vi "SRV_Write-Read Package.vi"(6 "Method":T2, 7 "parameters":T1={"bytes to read"=2000, "msec pause"=0, "msec timeout"=1000}, 8 "error in":errorcluster, 9 "listing in":string, 10 "data in":string, 11 "connection ID in":refnum<k5>) -> (0 "error out":errorcluster, 1 "listing out":string, 2 "data out":string, 3 "connection ID":refnum<k5>)   [LabVIEW 2014]
doc: "Modified for Benilde St. Margaret's School - Tim Jump\nBy Doug Schmertman - Logic PD\nCopyright 2012"
uses:
  SRV_Package Methods.ctl
  SRV_TCP Settings.ctl
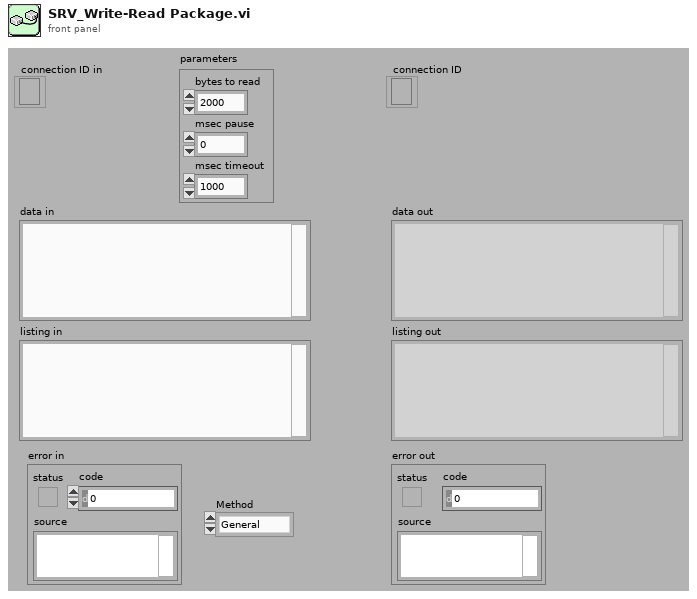
[diagram p1: front panel]
types:
  T1 = cluster{"bytes to read":i32, "msec pause":u32, "msec timeout":i32}
  T2 = typedef "SRV_Package Methods.ctl" = enum16{"General", "Standard", "CRLF", "Image", "HTML"}
  T3 = typedef "SRV_TCP Settings.ctl" = cluster{"Method":T2, "bytes to read":i32, "timeout ms (1000)":i32}
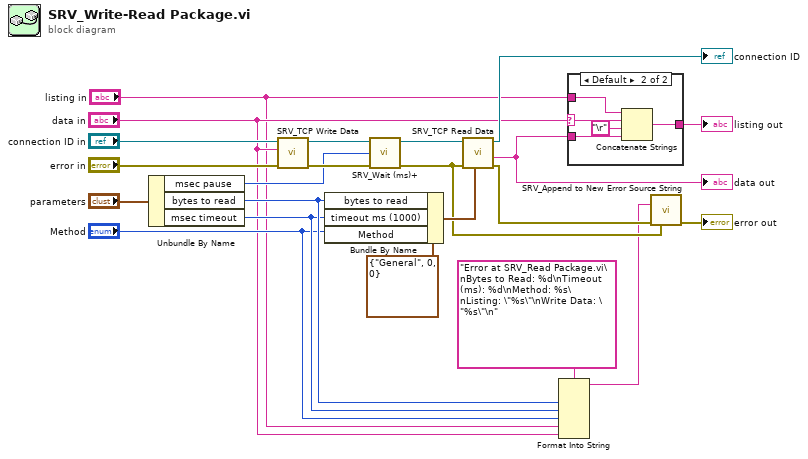
[diagram p0: block diagram]
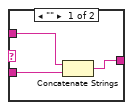
[diagram p2: hidden frame]
diagram:
  n1 = Unbundle By Name("parameters") -> ("msec pause"=w12:u32, "bytes to read"=w6:i32, "msec timeout"=w5:i32)
  n2 = call "SRV_TCP Write Data.vi"("error in"="error in", "data in"="data in", "connection ID"="connection ID in") -> ("error out"=w13:errorcluster, "connection ID out"=w14:refnum<k5>)  [unwired: 6 in, 1 out]
  n3 = Bundle By Name(cluster=T3 {"Method"=enum."General", "bytes to read"=0, "timeout ms (1000)"=0} ("TCP Settings"), "bytes to read"=w6, "timeout ms (1000)"=w5, "Method"="Method") -> (w15:T3)
  n4 = call "SRV_Wait (ms)+.vi"("milliseconds to wait"=w12, "error in (no error)"=w13) -> ("error out"=w10:errorcluster)  [unwired: 12 in, 1 out]
  n5 = call "SRV_TCP Read Data.vi"("TCP Settings"=w15, "error in"=w10, "connection ID in"=w14) -> ("error out"=w9:errorcluster, "data out"=w16:string, "connection ID"=→"connection ID":refnum<k5>)  [unwired: 2 in, 1 out]
  "data out" <- w16
  n6 = Format Into String(format string="Error at SRV_Read Package.vi\nBytes to Read: %d\nTimeout (ms): %d\nMethod: %s\nListing: \"%s\"\nWrite Data: \"%s\"\n", w6, w5, "Method", "listing in", "data in") -> (resulting string=w3:string)  [unwired: 2 in, 1 out]
  n7 = case shown="Default" "data in" {
    selector: "data in" -> [_ w25]
    tunnel: [w22 w29] -> w21
    tunnel: "listing in" -> [w24 w27]
    tunnel: w16 -> [w23 w26]
    frame "" {
      n8 = Concatenate Strings(w24, w23) -> (w22:string)
    }
    frame Default {
      n9 = Concatenate Strings(w27, w25, "\r", w26) -> (w29:string)
    }
  }
  "listing out" <- w21
  n10 = call "SRV_Append to New Error Source String.vi"("Message String to append"=w3, "Error In (no error)"=w9, "Previous Error In (no error)"=w10) -> ("error out"=→"error out":errorcluster)  [unwired: 12 in]
